vi "get_Paired_Wire_Index.vi"(8 "error in (no error)":errorcluster, 11 "CtrlLine in":refnum<class "CtrlLine.lvclass">) -> (0 "error out":errorcluster, 2 "Paired Wire Index":i32, 3 "CtrlLine out":refnum<class "CtrlLine.lvclass">)   [LabVIEW 2020, in "CtrlLine.lvclass"]
uses:
  CtrlLine.lvclass
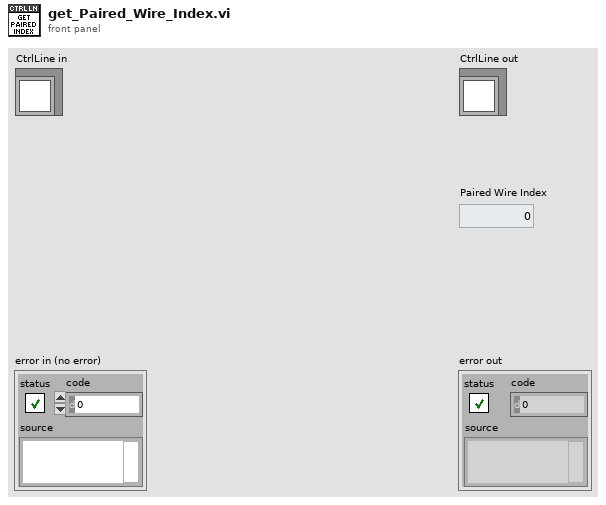
[diagram p1: front panel]
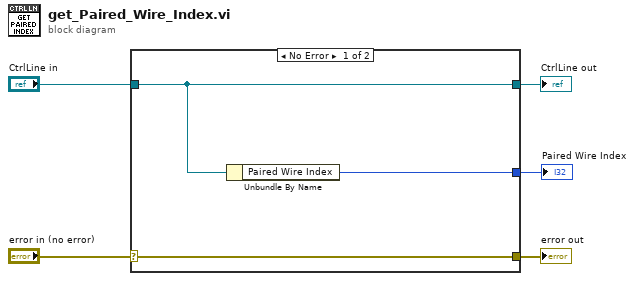
[diagram p0: block diagram]
diagram:
  n1 = case shown="No Error" "error in (no error)" {
    selector: "error in (no error)" -> [w8 w9]
    tunnel: [w8 w9] -> w4
    tunnel: [w7 w10] -> w2
    tunnel: "CtrlLine in" -> [w7 w10]
    tunnel: [w6 _] -> w1
    frame No Error {
      n2 = Unbundle By Name(w7) -> ("Paired Wire Index"=w6:i16)
    }
    frame Error {
    }
  }
  "error out" <- w4
  "CtrlLine out" <- w2
  "Paired Wire Index" <- w1
